vi "图片分析.vi"() -> ()   [LabVIEW 2018]
uses:
  <vilib>/vision/NI_Vision_Development_Module.lvlib
panel:
  in  "样本图路径.bmp":path
  in  "停止按钮":bool
  in  "颜色阈值":T1(radio)
  out "阈值图像":T2(plugin-control)
  out "源图像":T2(plugin-control)
  in  "Test Image":enum32{"Image1", "Image2"}(radio)
  in  "Blue or Luminance":cluster{i32, i32}(slide)={0, 5} scale=0.0..255.0
  in  "Green or Saturation":cluster{i32, i32}(slide)={0, 5} scale=0.0..255.0
  in  "Red or Hue":cluster{i32, i32}(slide)={0, 5} scale=0.0..255.0
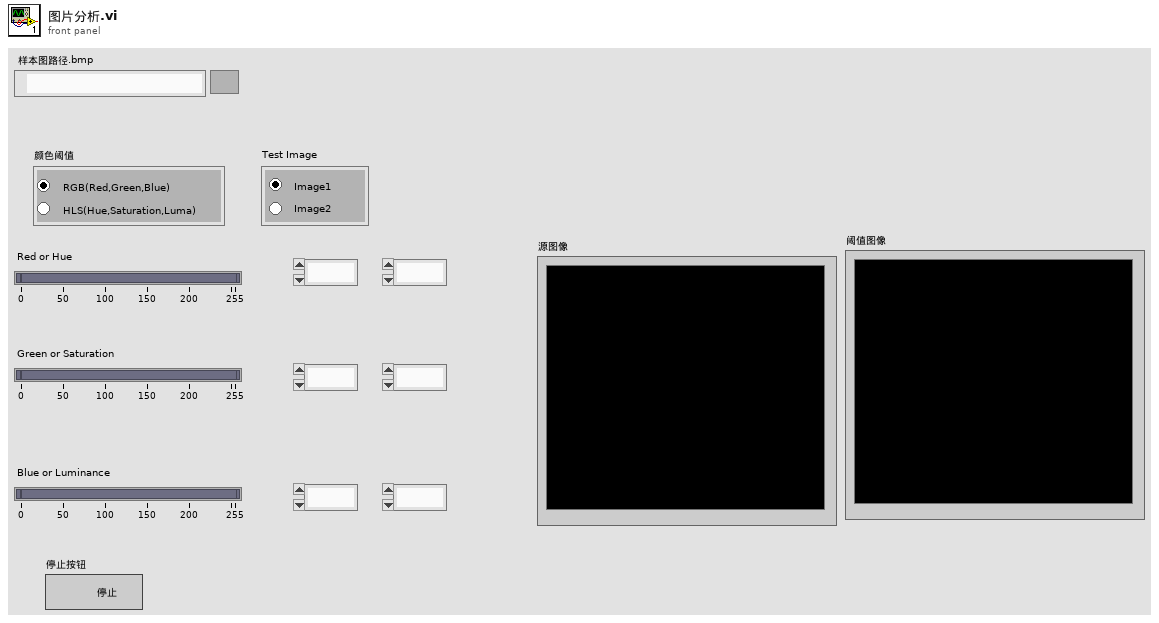
[diagram p1: front panel]
types:
  T1 = enum32{"RGB(Red,Green,Blue)", "HLS(Hue,Saturation,Luma)"}
  T2 = typedef "IMAQ Image.ctl" = refnum<image>
  T3 = typedef "Image Type" = u32
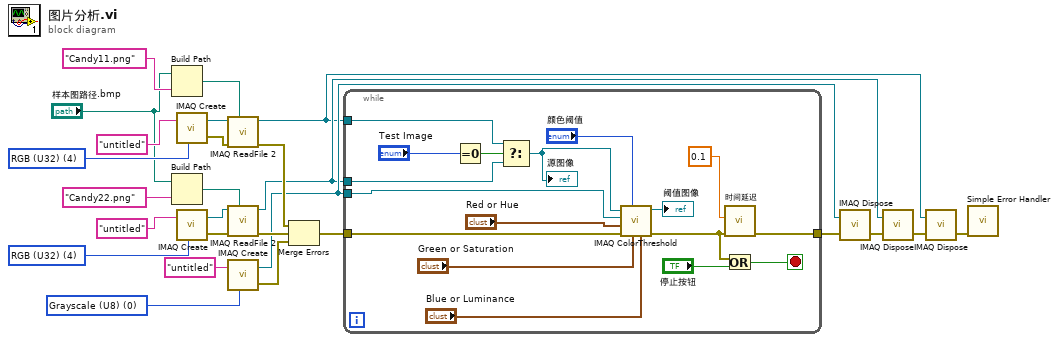
[diagram p0: block diagram]
diagram:
  w21 = T3 0 items=["Grayscale (U8)", "Grayscale (I16)", "Grayscale (SGL)", "Complex (CSG)", "RGB (U32)", "HSL (U32)", "RGB (U64)", "Grayscale (U16)"] ("Image Type")
  w23 = T3 4 items=["Grayscale (U8)", "Grayscale (I16)", "Grayscale (SGL)", "Complex (CSG)", "RGB (U32)", "HSL (U32)", "RGB (U64)", "Grayscale (U16)"] ("Image Type")
  w25 = T3 4 items=["Grayscale (U8)", "Grayscale (I16)", "Grayscale (SGL)", "Complex (CSG)", "RGB (U32)", "HSL (U32)", "RGB (U64)", "Grayscale (U16)"] ("Image Type")
  n1 = Build Path(base path="样本图路径.bmp", name or relative path="Candy11.png" ("名称或相对路径")) -> (appended path=w14:path)
  n2 = Build Path(base path="样本图路径.bmp", name or relative path="Candy22.png" ("名称或相对路径")) -> (appended path=w13:path)
  n3 = call "IMAQ Create"("Image Name"="untitled", "Image Type"=w25) -> ("New Image"=w19:T2, "error out"=w18:errorcluster)  [unwired: 3 in]
  n4 = call "IMAQ Create"("Image Name"="untitled", "Image Type"=w23) -> ("New Image"=w17:T2, "error out"=w16:errorcluster)  [unwired: 3 in]
  n5 = call "IMAQ ReadFile 2"("File Path"=w14, "error in (no error)"=w18, "Image"=w19) -> ("error out"=w10:errorcluster, "Image Out"=w3:T2)  [unwired: 4 in, 3 out]
  n6 = call "IMAQ ReadFile 2"("File Path"=w13, "error in (no error)"=w16, "Image"=w17) -> ("error out"=w11:errorcluster, "Image Out"=w4:T2)  [unwired: 4 in, 3 out]
  n7 = call "IMAQ Create"("Image Name"="untitled", "Image Type"=w21) -> ("New Image"=w5:T2, "error out"=w12:errorcluster)  [unwired: 3 in]
  n8 = Merge Errors(w10, w11, w12) -> (w9:errorcluster)
  n9 = while {
    tunnel: w9 -> [w40]
    tunnel: w3 -> [w35]
    tunnel: w4 -> [w36]
    tunnel: w5 -> [w39]
    tunnel: [w27] -> w8
    stop <- w28 stop-if-true
    n10 = Equal To 0?(x="Test Image") -> (x = 0?=w38:bool)
    n11 = Select(t=w35, s=w38, f=w36) -> (s? t:f=w33:T2)
    "源图像" <- w33
    n12 = call "IMAQ ColorThreshold"("Blue or Luma or Val or Inten Range"="Blue or Luminance", "Green or Sat Range"="Green or Saturation", "Color Mode"="颜色阈值", "error in (no error)"=w40, "Red or Hue Range"="Red or Hue", "Image Dst"=w39, "Image Src"=w33) -> ("error out"=w29:errorcluster, "Image Dst Out"=→"阈值图像":T2)  [unwired: 3 in]
    n13 = call "时间延迟"("error in (no error)"=w29, "Delay Time (s)"=0.1) -> ("error out"=w27:errorcluster)  [unwired: 9 in]
    n14 = Or(x=w29, y="停止按钮") -> (x .or. y?=w28:bool)
  }
  n15 = call "IMAQ Dispose"("Image"=w5, "error in (no error)"=w8) -> ("error out"=w7:errorcluster)  [unwired: 4 in]
  n16 = call "IMAQ Dispose"("Image"=w4, "error in (no error)"=w7) -> ("error out"=w6:errorcluster)  [unwired: 4 in]
  n17 = call "IMAQ Dispose"("Image"=w3, "error in (no error)"=w6) -> ("error out"=w1:errorcluster)  [unwired: 4 in]
  n18 = call <vilib>:"Simple Error Handler.vi"("error in (no error)"=w1) -> ()  [unwired: 4 in, 5 out]
